vi "save average to file.vi"(8 "error in (no error)":errorcluster, 10 "filename":string, 11 "LineCCD in":refnum<class "LineCCD.lvclass">) -> (0 "error out":errorcluster, 3 "LineCCD out":refnum<class "LineCCD.lvclass">)   [LabVIEW 2012, in "LineCCD.lvclass"]
uses:
  LineCCD.lvclass
  LineCCD.lvclass/LineCCD.ctl
  <vilib>/Utility/file.llb/Write To Spreadsheet File (DBL).vi
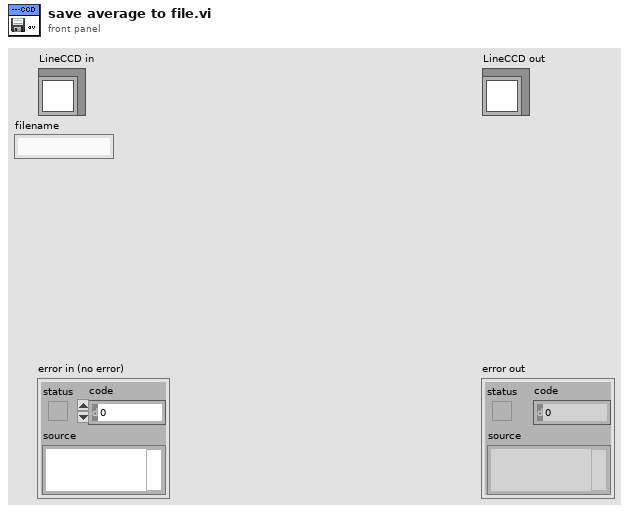
[diagram p1: front panel]
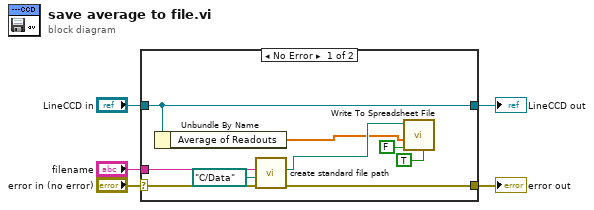
[diagram p0: block diagram]
diagram:
  n1 = case shown="No Error" "error in (no error)" {
    selector: "error in (no error)" -> [w13 w16]
    tunnel: [w12 w16] -> w4
    tunnel: [w14 w15] -> w2
    tunnel: "LineCCD in" -> [w14 w15]
    tunnel: "filename" -> [w10 _]
    frame No Error {
      n2 = Unbundle By Name(w14) -> ("Average of Readouts"=w6:dbl[])
      n3 = call "create standard file path.vi"("error in (no error)"=w13, "base path"=path "C:/Data", "filename"=w10) -> ("error out"=w12:errorcluster, "complete\n path"=w7:path)  [unwired: 5 in]
      n4 = call-poly <vilib>:"Write To Spreadsheet File.vi"("transpose? (no:F)"=TRUE, "append to file? (new file:F)"=FALSE, "1D data"=w6, "file path (dialog if empty)"=w7) -> ()  [unwired: 4 in, 1 out]
    }
    frame Error {
    }
  }
  "error out" <- w4
  "LineCCD out" <- w2
